vi "facade.vi"(0 "Data In":T4, 2 "Display State In":T2, 3 "Container State":T3) -> (6 "Data Out":T4, 7 "Display State Out":T2, 8 "Action":T1)   [LabVIEW 2010, in "XSettings.xctl"]
uses:
  XSettings.xctl
  data.ctl
  classes/GenericComponent/GenericComponent/GenericComponent.lvclass
  <vilib>/_xctls/Container State.ctl
  state.ctl
  <vilib>/_xctls/Action.ctl
  <vilib>/_xctls/XControlSupport.lvlib
panel:
  in  "loadButton":bool
  in  "saveButton":bool
  in  "settings":string(combo)
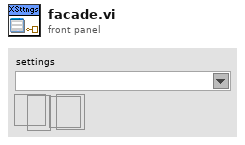
[diagram p1: front panel]
types:
  T1 = typedef "XControlSupport.lvlib/Action.ctl" = cluster{"Data Changed?":bool, "State Changed?":bool, "Action Name":string}
  T2 = typedef "XSettings.xctl/state.ctl" = cluster{"error":errorcluster, "user-defined?":bool, "control refs":cluster{"settings combo":refnum<vi>}}
  T3 = typedef "XControlSupport.lvlib/Container State.ctl" = cluster{"Indicator?":bool, "Run Mode?":bool, " Refnum":refnum<vi>}
  T4 = typedef "XSettings.xctl/data.ctl" = refnum<class "GenericComponent.lvclass">
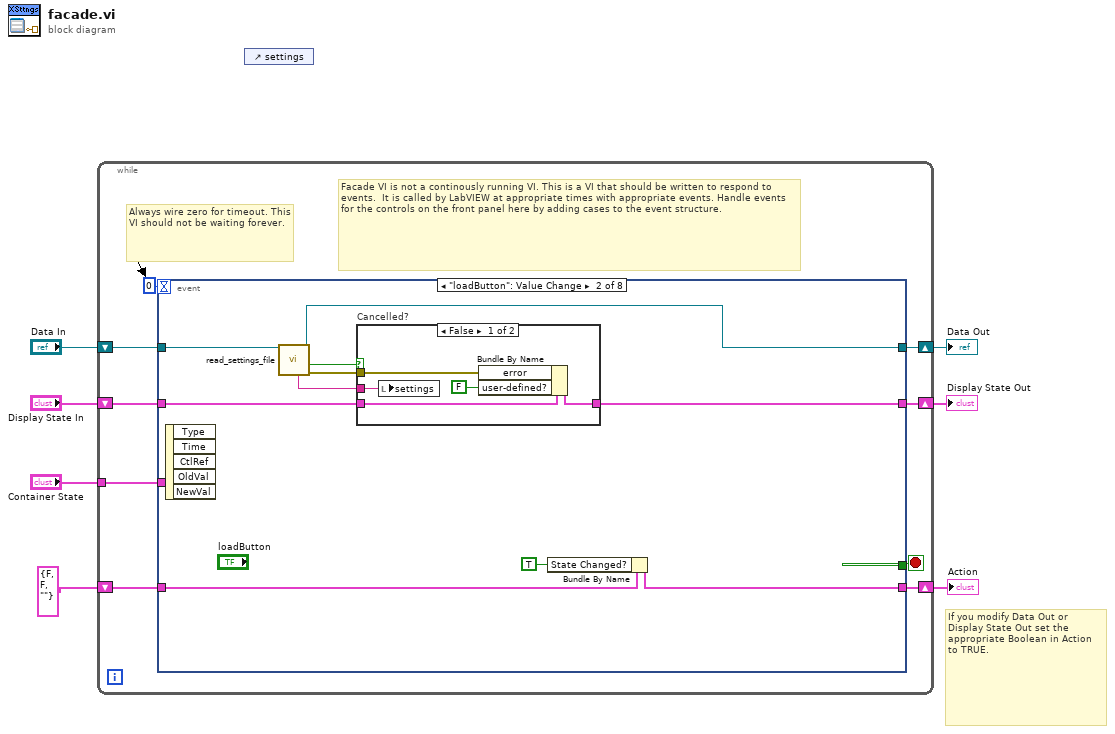
[diagram p0: block diagram]
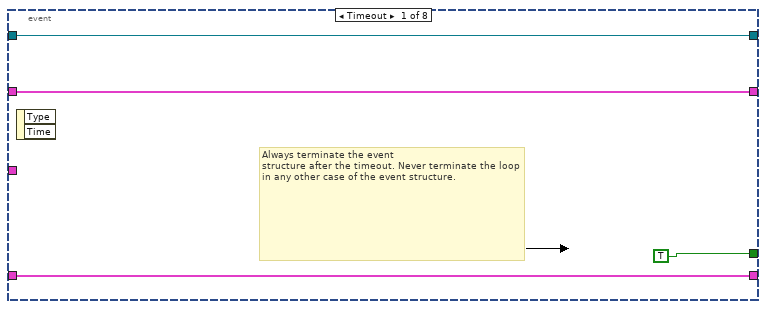
[diagram p2: hidden frame]
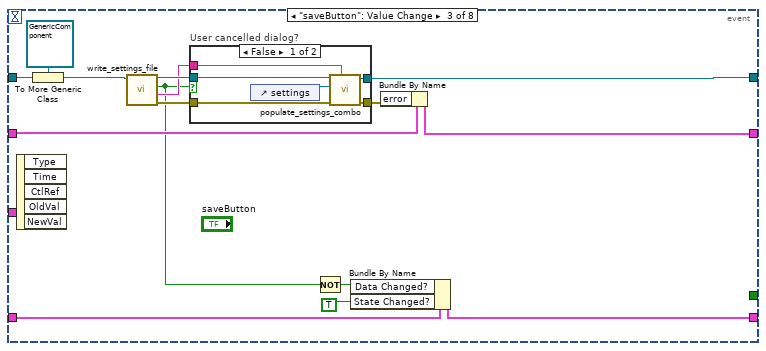
[diagram p4: hidden frame]
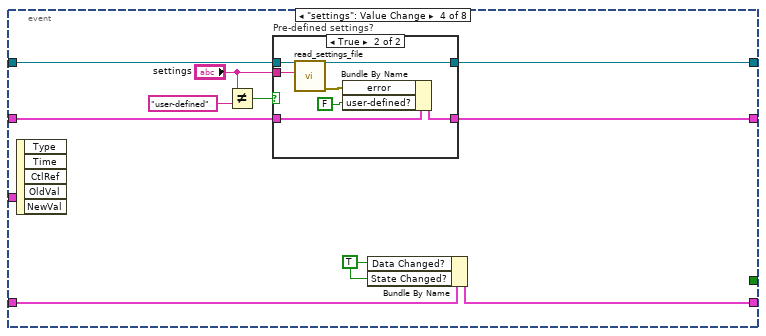
[diagram p6: hidden frame]
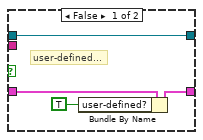
[diagram p7: hidden frame]
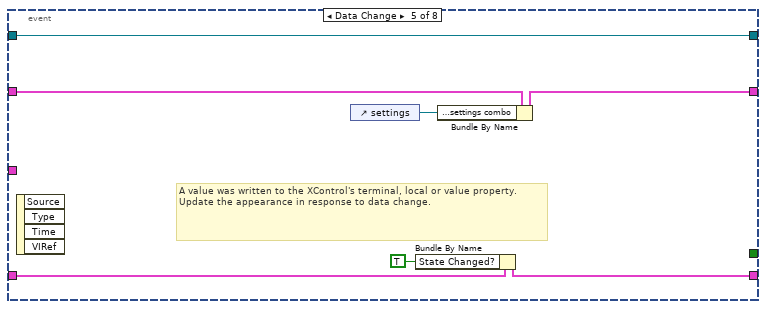
[diagram p8: hidden frame]
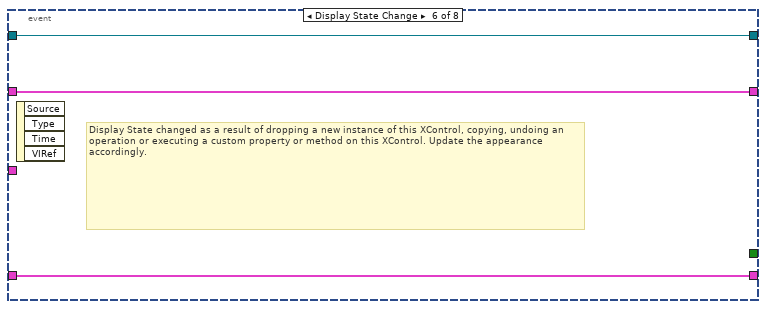
[diagram p9: hidden frame]
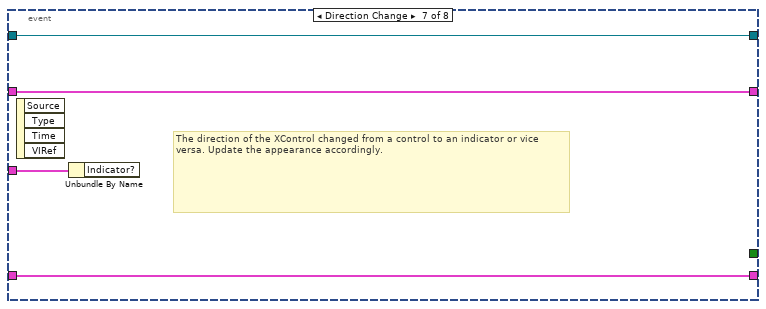
[diagram p10: hidden frame]
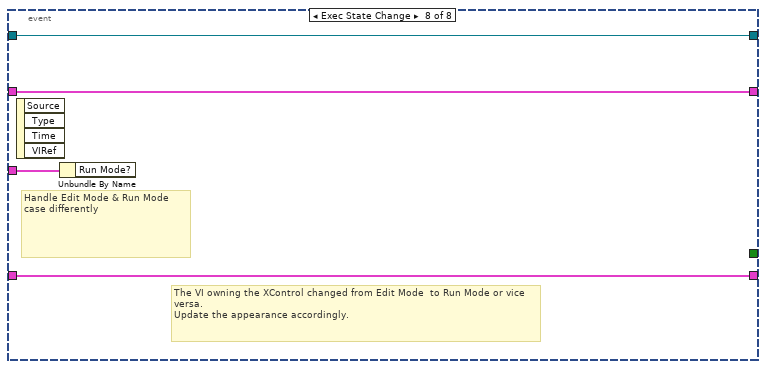
[diagram p11: hidden frame]
diagram:
  # "If you modify Data Out or\nDisplay State Out set the\nappropriate Boolean in Action\nto TRUE."
  n1 = while {
    shift-right: [w15] -> w4
    shift-left: "Display State In" -> [w16]
    tunnel: "Container State" -> [w12]
    shift-right: [w10] -> w7
    shift-left: "Data In" -> [w11]
    shift-right: [w8] -> w2
    shift-left: T1 {"Data Changed?"=FALSE, "State Changed?"=FALSE, "Action Name"=""} ("Action") -> [w9]
    stop <- w14 stop-if-true
    # "Facade VI is not a continously running VI. This is a VI that should be written to respond to events.  It is called by LabVIEW at appropriate times with appropriate events. Handle events for the controls on the front panel here by adding cases to the event structure."
    # "Always wire zero for timeout. This\nVI should not be waiting forever."
    n2 = event shown="[1] \"loadButton\": Value Change" {
      selector: _ -> [_ _ _ _ _ _ _ _]
      dyn-events: _ -> [_ _ _ _ _ _ _ _]
      timeout: 0 -> [_ _ _ _ _ _ _ _]
      tunnel: w16 -> [w18 w28 w51 w67 w86 w90 w93 w95]
      tunnel: [w18 w27 w50 w66 w87 w90 w93 w95] -> w15
      tunnel: [TRUE _ _ _ _ _ _ _] -> w14
      tunnel: w12 -> [_ _ _ _ _ _ w94 w98]
      tunnel: w11 -> [w17 w30 w39 w69 w81 w89 w92 w96]
      tunnel: [w17 w21 w42 w68 w81 w89 w92 w96] -> w10
      tunnel: [w19 w24 w47 w64 w82 w88 w91 w97] -> w8
      tunnel: w9 -> [w19 w25 w48 w65 w83 w88 w91 w97]
      event Timeout {
        # "Always terminate the event\nstructure after the timeout. Never terminate the loop in any other case of the event structure."
        n3 = event-data() -> ()  [unwired: 1 in, 2 out]
      }
      event "loadButton": Value Change {
        n4 = event-data() -> ()  [unwired: 1 in, 5 out]
        n5 = call-dynamic "read_settings_file.vi"("GenericComponent in"=w30) -> ("error out"=w29:errorcluster, "cancelled?"=w22:bool, "GenericComponent out"=w21:T4, "name"=w23:string)  [unwired: 6 in, 1 out]
        n6 = case "Cancelled?" shown="False" w22 {
          tunnel: w29 -> [w35 _]
          tunnel: w28 -> [w34 w36]
          tunnel: [w33 w36] -> w27
          tunnel: w23 -> [w31 _]
          frame False {
            n7 = local write "settings"(w31) -> ()
            n8 = Bundle By Name(cluster=w34, "error"=w35, "user-defined?"=FALSE) -> (w33:T2)
          }
          frame True {
          }
        }
        n9 = Bundle By Name(cluster=w25, "State Changed?"=TRUE) -> (w24:T1)
      }
      event "saveButton": Value Change {
        n10 = event-data() -> ()  [unwired: 1 in, 5 out]
        n11 = To More Generic Class(target class=refnum<class "GenericComponent.lvclass"> refnum ("GenericPlugin in"), reference=w39) -> (generic class reference=w37:refnum<class "GenericComponent.lvclass">)
        n12 = call-dynamic "write_settings_file.vi"("GenericPlugin in"=w37) -> ("error out"=w45:errorcluster, "settings name (wihout \".xml\" file ending)"=w41:string, "cancelled?"=w40:bool, "GenericPlugin out"=w43:refnum<class "GenericComponent.lvclass">)  [unwired: 7 in]
        n13 = case "User cancelled dialog?" shown="False" w40 {
          tunnel: w45 -> [w56 w59]
          tunnel: [w55 w59] -> w44
          tunnel: w43 -> [w54 w58]
          tunnel: [w53 w58] -> w42
          tunnel: w41 -> [w52 _]
          frame False {
            n14 = control-ref of="settings"() -> (w57:refnum<vi>)
            n15 = call-dynamic "populate_settings_combo.vi"("force settings"=w52, "error in (no error)"=w56, "combo box ref"=w57, "GenericPlugin in"=w54) -> ("error out"=w55:errorcluster, "GenericPlugin out"=w53:refnum<class "GenericComponent.lvclass">)  [unwired: 6 in]
          }
          frame True {
          }
        }
        n16 = Not(x=w40) -> (.not. x?=w49:bool)
        n17 = Bundle By Name(cluster=w48, "Data Changed?"=w49, "State Changed?"=TRUE) -> (w47:T1)
        n18 = Bundle By Name(cluster=w51, "error"=w44) -> (w50:T2)
      }
      event "settings": Value Change {
        w63 = TRUE ("Data Changed?")
        n19 = event-data() -> ()  [unwired: 1 in, 5 out]
        n20 = Not Equal?(x="settings", y="user-defined") -> (x != y?=w60:bool)
        n21 = case "Pre-defined settings?" shown="True" w60 {
          tunnel: w69 -> [w73 w80]
          tunnel: [w73 w79] -> w68
          tunnel: w67 -> [w72 w78]
          tunnel: [w71 w77] -> w66
          tunnel: "settings" -> [_ w75]
          frame False {
            # "user-defined..."
            n22 = Bundle By Name(cluster=w72, "user-defined?"=TRUE) -> (w71:T2)
          }
          frame True {
            n23 = call-dynamic "read_settings_file.vi"("settings name"=w75, "GenericComponent in"=w80) -> ("error out"=w76:errorcluster, "GenericComponent out"=w79:T4)  [unwired: 5 in, 3 out]
            n24 = Bundle By Name(cluster=w78, "error"=w76, "user-defined?"=FALSE) -> (w77:T2)
          }
        }
        n25 = Bundle By Name(cluster=w65, "Data Changed?"=w63, "State Changed?"=w63) -> (w64:T1)
      }
      event Data Change {
        # "A value was written to the XControl's terminal, local or value property.\nUpdate the appearance in response to data change."
        n26 = event-data() -> ()  [unwired: 1 in, 4 out]
        n27 = control-ref of="settings"() -> (w85:refnum<vi>)
        n28 = Bundle By Name(cluster=w83, "State Changed?"=TRUE ("Data Changed?")) -> (w82:T1)
        n29 = Bundle By Name(cluster=w86, "control refs.settings combo"=w85) -> (w87:T2)
      }
      event Display State Change {
        # "Display State changed as a result of dropping a new instance of this XControl, copying, undoing an operation or executing a custom property or method on this XControl. Update the appearance accordingly."
        n30 = event-data() -> ()  [unwired: 1 in, 4 out]
      }
      event Direction Change {
        # "The direction of the XControl changed from a control to an indicator or vice versa. Update the appearance accordingly."
        n31 = event-data() -> ()  [unwired: 1 in, 4 out]
        n32 = Unbundle By Name(w94) -> ()  [unwired: 1 out]
      }
      event Exec State Change {
        # "The VI owning the XControl changed from Edit Mode  to Run Mode or vice versa.\nUpdate the appearance accordingly."
        # "Handle Edit Mode & Run Mode\ncase differently"
        n33 = event-data() -> ()  [unwired: 1 in, 4 out]
        n34 = Unbundle By Name(w98) -> ()  [unwired: 1 out]
      }
    }
  }
  "Display State Out" <- w4
  "Data Out" <- w7
  "Action" <- w2
  n35 = control-ref of="settings"() -> ()  [unwired: 1 out]
